vi "Apply Column Setup After Binding.vi"(8 "error in (no error)":errorcluster, 11 "DataGridView in":refnum<class "DataGridView.lvclass">) -> (0 "error out":errorcluster, 3 "DataGridView out":refnum<class "DataGridView.lvclass">)   [LabVIEW 2014, in "DataGridView.lvclass"]
doc: "This is called after populating the datagridview (via binding its DataTable) so that the custom datatypes can be setup for the columns that require it. This is only needed if you are using <B>Buttons</B> or <B>Combos</B> as all other types are completely automatic."
uses:
  DataGridView.lvclass
  DataGridView.lvclass/DataGridView.ctl
  System.Windows.Forms
  GridColumn/GridColumn.lvclass/GridColumn.ctl
  GridColumn/Read Params.vi
  GridColumn/Read Name.vi
  GridColumn/Read AutoSizeMode.vi
  GridColumn/Read FillWeight.vi
  GridColumn/Read datatype.vi
  GridColumn/GridColumn.lvclass
  <vilib>/Prolucid Technologies/PLT Common Functions/PLT Common Functions.lvlib
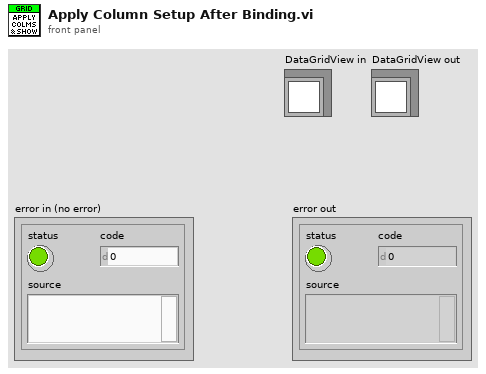
[diagram p1: front panel]
types:
  T1 = enum16{"string", "image", "check", "numeric", "timestamp", "button", "combo"}
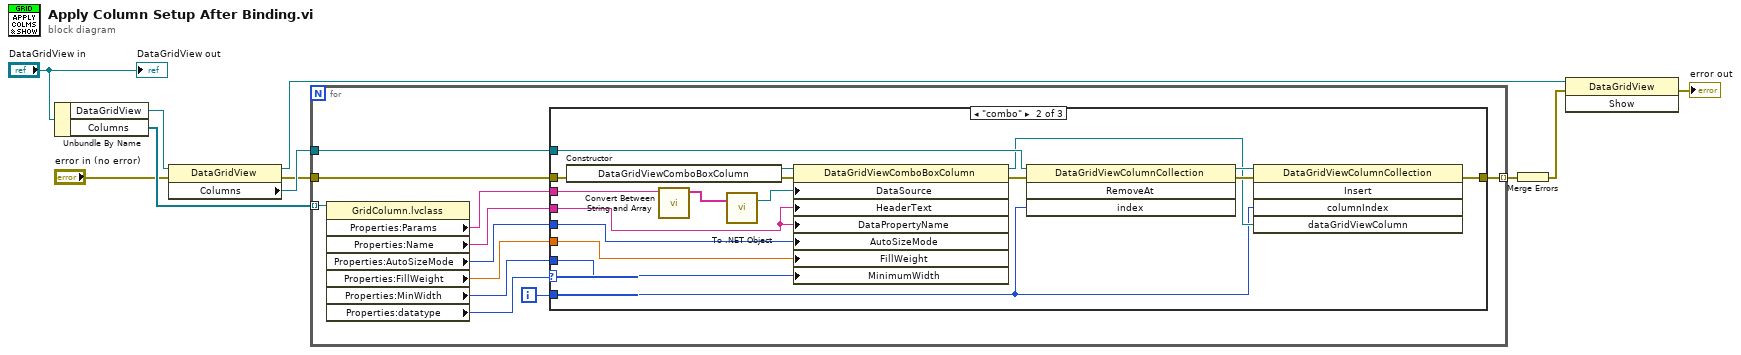
[diagram p0: block diagram]
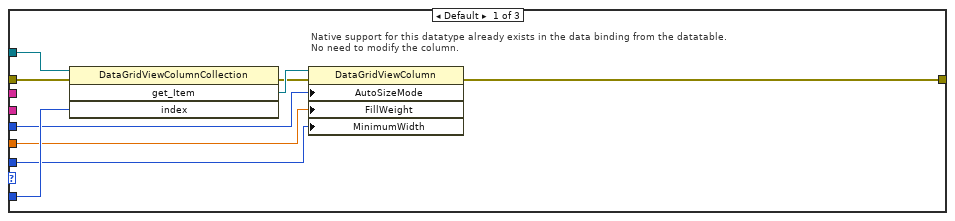
[diagram p2: hidden frame]
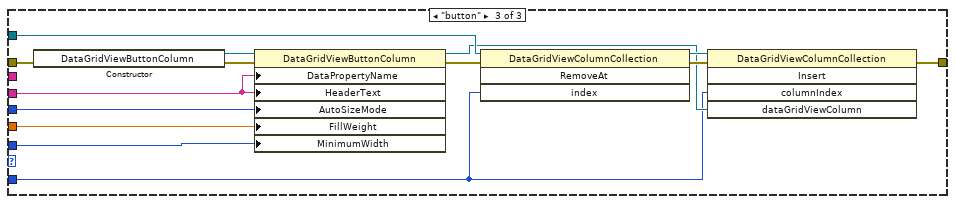
[diagram p3: hidden frame]
diagram:
  n1 = Unbundle By Name("DataGridView in") -> ("DataGridView"=w7:refnum<k24>, "Columns"=w8:refnum<class "GridColumn.lvclass">[])
  n2 = property class="DataGridView"(reference=w7, error in="error in (no error)") -> (reference out=w2:refnum<k24>, error out=w3:errorcluster, "Columns"=w6:refnum<k24>)
  n3 = for {
    tunnel: w6 -> [w21]
    tunnel: [w20] -> w9 mode=indexing
    tunnel: w8 -> [w17] mode=indexing
    tunnel: w3 -> [w18]
    i -> [w19]
    n4 = property class="GridColumn.lvclass"(reference=w17) -> ("Properties:Params"=w16:string, "Properties:Name"=w15:string, "Properties:AutoSizeMode"=w14:i32, "Properties:FillWeight"=w11:sgl, "Properties:MinWidth"=w13:u32, "Properties:datatype"=w12:T1)  [unwired: 1 in, 2 out]
    n5 = case shown="\"combo\"" w12 {
      tunnel: w21 -> [w30 w45 w59]
      tunnel: [w22 w41 w55] -> w20
      tunnel: w19 -> [w29 w38 w53]
      tunnel: w15 -> [_ w36 w52]
      tunnel: w16 -> [_ w32 _]
      tunnel: w13 -> [w24 w33 w51]
      tunnel: w11 -> [w25 w34 w50]
      tunnel: w14 -> [w26 w35 w49]
      tunnel: w18 -> [w23 w31 w48]
      frame Default {
        # "Native support for this datatype already exists in the data binding from the datatable.\nNo need to modify the column."
        n6 = invoke class="DataGridViewColumnCollection" method="get_Item"(reference=w30, error in=w23, "index"=w29) -> (error out=w27:errorcluster, "get_Item"=w28:refnum<k24>)  [unwired: 1 in, 2 out]
        n7 = property class="DataGridViewColumn"(reference=w28, error in=w27, "AutoSizeMode"=w26, "FillWeight"=w25, "MinimumWidth"=w24) -> (error out=w22:errorcluster)  [unwired: 1 out]
      }
      frame "combo" {
        n8 = constructor class="DataGridViewComboBoxColumn"(error in=w31) -> (reference out=w47:refnum<k24>, error out=w46:errorcluster)  [unwired: 2 in, 1 out]
        n9 = call <vilib>:"Convert Between String and Array.vi"("String"=w32) -> ("String Array"=w37:string[])  [unwired: 9 in, 1 out]
        n10 = call <vilib>:"To .NET Object.vi"("anything"=w37) -> (".NET object"=w40:refnum<k24>)  [unwired: 1 in, 1 out]
        n11 = property class="DataGridViewComboBoxColumn"(reference=w47, error in=w46, "DataSource"=w40, "HeaderText"=w36, "DataPropertyName"=w36, "AutoSizeMode"=w35, "FillWeight"=w34, "MinimumWidth"=w33) -> (reference out=w42:refnum<k24>, error out=w39:errorcluster)
        n12 = invoke class="DataGridViewColumnCollection" method="RemoveAt"(reference=w45, error in=w39, "index"=w38) -> (reference out=w43:refnum<k24>, error out=w44:errorcluster)  [unwired: 1 in, 2 out]
        n13 = invoke class="DataGridViewColumnCollection" method="Insert"(reference=w43, error in=w44, "columnIndex"=w38, "dataGridViewColumn"=w42) -> (error out=w41:errorcluster)  [unwired: 1 in, 4 out]
      }
      frame "button" {
        n14 = constructor class="DataGridViewButtonColumn"(error in=w48) -> (reference out=w61:refnum<k24>, error out=w60:errorcluster)  [unwired: 2 in, 1 out]
        n15 = property class="DataGridViewButtonColumn"(reference=w61, error in=w60, "DataPropertyName"=w52, "HeaderText"=w52, "AutoSizeMode"=w49, "FillWeight"=w50, "MinimumWidth"=w51) -> (reference out=w56:refnum<k24>, error out=w54:errorcluster)
        n16 = invoke class="DataGridViewColumnCollection" method="RemoveAt"(reference=w59, error in=w54, "index"=w53) -> (reference out=w57:refnum<k24>, error out=w58:errorcluster)  [unwired: 1 in, 2 out]
        n17 = invoke class="DataGridViewColumnCollection" method="Insert"(reference=w57, error in=w58, "columnIndex"=w53, "dataGridViewColumn"=w56) -> (error out=w55:errorcluster)  [unwired: 1 in, 4 out]
      }
    }
  }
  n18 = Merge Errors(w9) -> (w1:errorcluster)
  n19 = invoke class="DataGridView" method="Show"(reference=w2, error in=w1) -> (error out=→"error out":errorcluster)  [unwired: 1 in, 2 out]
  "DataGridView out" <- "DataGridView in"
